vi "MDrive-Test.vi"() -> ()   [LabVIEW 2011]
uses:
  <vilib>/Instr/_visa.llb/VISA Configure Serial Port (Instr).vi
panel:
  in  "baud rate":u32=9600
  out "Size":i32
  out "Received":string
  in  "Quit":bool
  in  "VISA resource name":refnum<visa-resource-name>
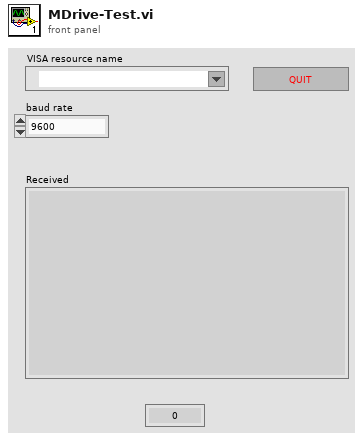
[diagram p1: front panel]
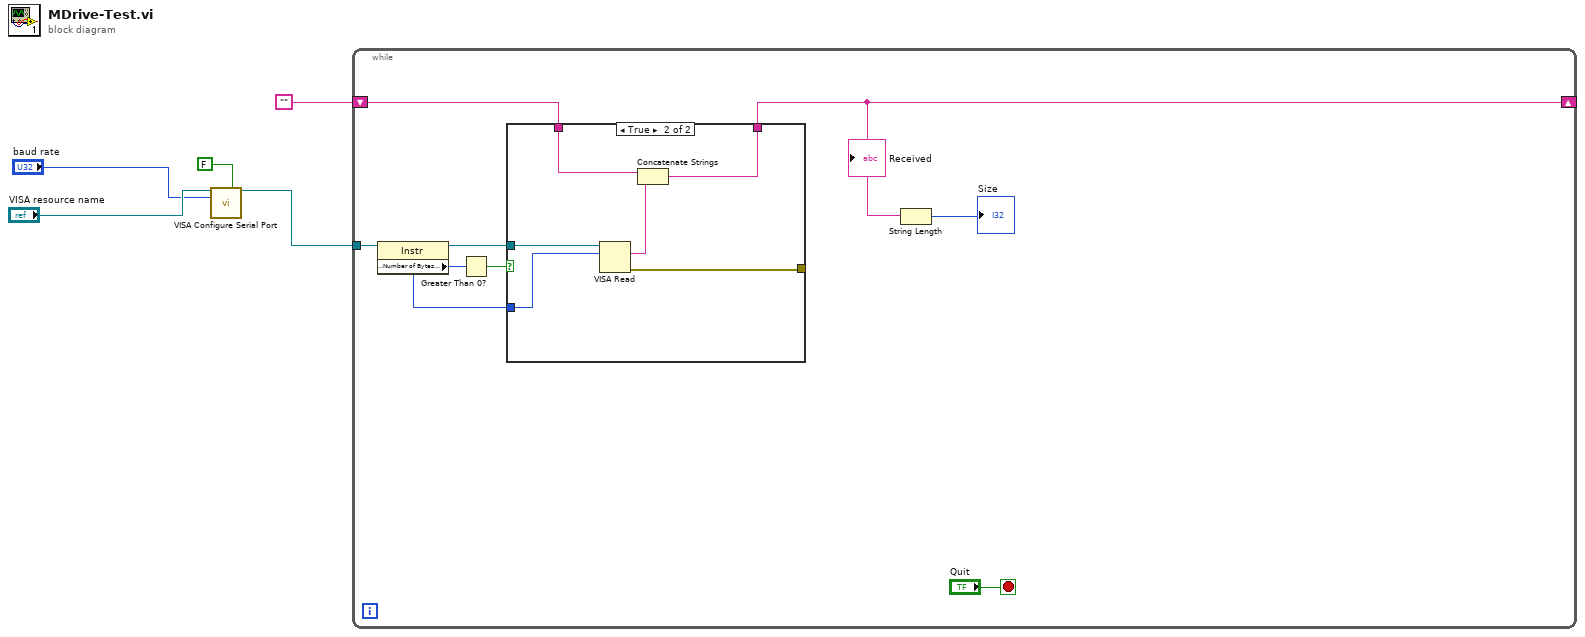
[diagram p0: block diagram]
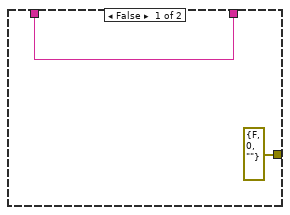
[diagram p2: hidden frame]
diagram:
  n1 = call-poly "VISA Configure Serial Port"("VISA resource name"="VISA resource name", "Enable Termination\nChar (T)"=FALSE ("Enable Termination\nChar (T)"), "baud rate (9600)"="baud rate") -> ("VISA resource name out"=w2:refnum<visa-resource-name>)  [unwired: 11 in, 1 out]
  n2 = while {
    tunnel: w2 -> [w13]
    shift-right: [w7] -> _
    shift-left: "" -> [w10]
    stop <- "Quit" stop-if-true
    n3 = property class="Instr"(reference=w13) -> (reference out=w9:refnum<visa-resource-name>, "Serial Settings:Number of Bytes at Serial Port"=w8:u32)  [unwired: 1 in, 1 out]
    n4 = Greater Than 0?(x=w8) -> (x > 0?=w11:bool)
    n5 = case shown="True" w11 {
      tunnel: w10 -> [w15 w21]
      tunnel: w9 -> [_ w20]
      tunnel: w8 -> [_ w19]
      tunnel: [w15 w17] -> w7
      tunnel: [errorcluster {"status"=FALSE, "code"=0, "source"=""} ("error out") w16] -> _
      frame False {
      }
      frame True {
        n6 = VISA Read(VISA resource name=w20, byte count=w19) -> (read buffer=w18:string, error out=w16:errorcluster)  [unwired: 1 in, 2 out]
        n7 = Concatenate Strings(w21, w18) -> (w17:string)
      }
    }
    "Received" <- w7
    n8 = String Length(string=w7) -> (length=→"Size":i32)
  }
